vi "Handle Command.vi"(8 "error in":errorcluster, 10 "Change Laser Enable in":refnum<class "Change Laser Enable State.lvclass">, 11 "Object In":refnum<class>) -> (0 "error out":errorcluster, 1 "Command Successful?":bool, 2 "Change Laser Enable out":refnum<class "Change Laser Enable State.lvclass">, 3 "Object Out":refnum<class>)   [LabVIEW 2014, in "ePAS Library.lvlib" / "Change Laser Enable State.lvclass"]
doc: "Abstract method for accomplishing the execution of a command directed to an instrument object on the wire."
uses:
  Change Laser Enable State.lvclass
  Instrument/ePAS.lvclass
  reusable/Instrument/Instrument.lvclass/Instrument.ctl
  Instrument/ePAS.lvclass/ePAS.ctl
  Change Laser Enable State.lvclass/Change Laser Enable State.ctl
  reusable/Instrument/Read Log Session.vi
  Instrument/Accessors/Read FPGA Session.vi
  reusable/Instrument/Read ExtCom.vi
  <vilib>/Utility/error.llb/Error Cluster From Error Code.vi
  <vilib>/rvi/errors/niLvFpgaAdjustHostInterfaceError.vi
  <userlib>/_Session Fwk/Session - Root.lvclass
  <vilib>/rvi/interface/nirviReadWriteControl/nirviReadWriteControl.xnode
  FPGA/R FPGA Ref.ctl
  FPGA Bitfiles/FPGAServerV2.lvbitx
  FPGA/Session/Exscalabar FPGA.lvclass
  ePAS Library.lvlib
  reusable/Session APIs/Session Log/System Log.lvclass
  NiFpgaLv.dll
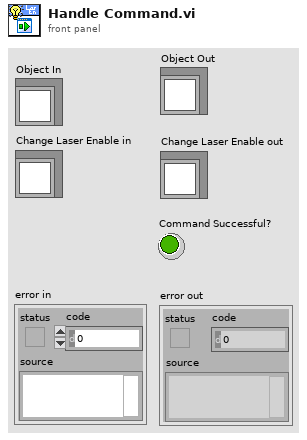
[diagram p1: front panel]
types:
  T1 = typedef "Session - Root.lvclass/Session Handle.ctl" = refnum<data-value>
  T2 = typedef "ePAS Library.lvlib/R FPGA Ref.ctl" = refnum<k20>
  T3 = cluster{"[0]":bool, "[1]":bool, "[2]":bool, "[3]":bool, "[4]":bool}
  T4 = cluster{"tag":string, "section":string, "data":variant}
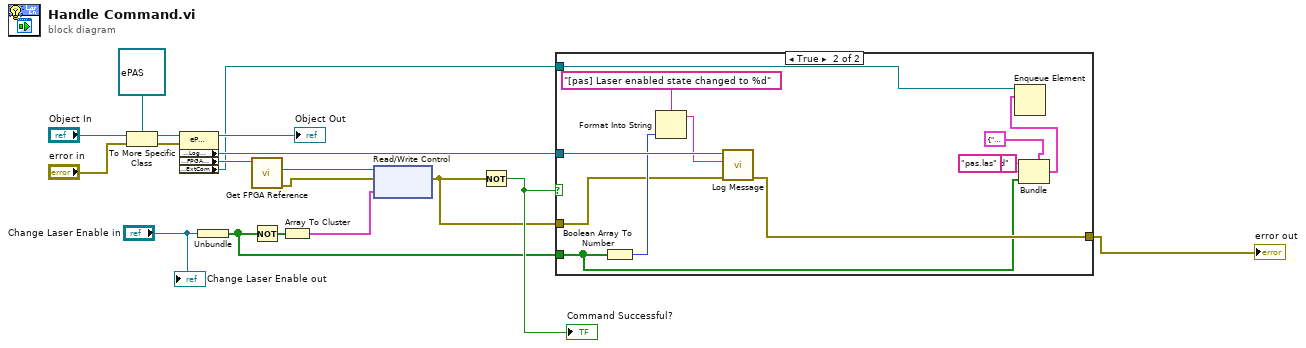
[diagram p0: block diagram]
diagram:
  n1 = To More Specific Class(target class=refnum<class "ePAS.lvclass"> refnum ("ePAS"), reference="Object In", error in="error in") -> (specific class reference=w4:refnum<class "ePAS.lvclass">, error out=w2:errorcluster)
  n2 = property class="ePAS"(reference=w4, error in=w2) -> (reference out=→"Object Out":refnum<class "ePAS.lvclass">, "Accessors:Log Session"=w10:T1, "Accessors:FPGA Session"=w3:T1, "Accessors:ExtCom"=w1:refnum<queue>)  [unwired: 1 out]
  n3 = Unbundle("Change Laser Enable in") -> (w8:bool[])
  n4 = call "Get FPGA Reference.vi"("Session In"=w3) -> ("error out"=w14:errorcluster, "Ex FPGA Ref"=w16:T2)  [unwired: 8 in, 1 out]
  n5 = Not(x=w8) -> (.not. x?=w9:bool[])
  n6 = Array To Cluster(array=w9) -> (cluster=w13:T3)
  n7 = xnode "Read/Write Control"("FPGA VI Reference In"=w16, "error in"=w14, "LaserEn"=w13) -> ("error out"=w7:errorcluster)  [unwired: 1 out]
  n8 = Not(x=w7) -> (.not. x?=w11:bool)
  "Command Successful?" <- w11
  n9 = case shown="True" w11 {
    tunnel: w10 -> [_ w31]
    tunnel: w8 -> [_ w25]
    tunnel: w7 -> [w19 w27]
    tunnel: [w19 w26] -> w6
    tunnel: w1 -> [_ w21]
    frame False {
    }
    frame True {
      n10 = Boolean Array To Number(Boolean array=w25) -> (number=w29:u32)
      n11 = Format Into String(format string="[pas] Laser enabled state changed to %d", w29) -> (resulting string=w28:string)  [unwired: 2 in, 1 out]
      n12 = call "Log Message.vi"("error in"=w27, "MSG In"=w28, "session in"=w31) -> ("error out"=w26:errorcluster)  [unwired: 7 in, 1 out]
      n13 = Bundle(cluster=T4 {"tag"="modulation", "section"="pas.las", "data"=variant} ("element"), "tag"="enabled", "section"="pas.las" ("tag"), "data"=w25) -> (w20:T4)
      n14 = Enqueue Element(queue=w21, element=w20) -> ()  [unwired: 2 in, 3 out]
    }
  }
  "error out" <- w6
  "Change Laser Enable out" <- "Change Laser Enable in"
